vi "DataGenerator.vi"() -> ()   [LabVIEW 2018, in "DataDisplay.lvlib"]
uses:
  DataDisplay.lvlib
  TypeDefine/DD_ChannelInfo.ctl
  <vilib>/measure/NI_MABase.lvlib
panel:
  in  "TrendPlot":bool
  in  "通道信息":T1[](array[typedef])=[{"名称"="位移1", "单位"="mm", "数据类型"=enum."Real", "趋势线"=enum."Y"}, {"名称"="位移2", "单位"="mm", "数据类型"=enum."Real", "趋势线"=enum."Y"}, {"名称"="力1", "单位"="mm", "数据类型"=enum."Real", "趋势线"=enum."N/A"}, {"名称"="力2", "单位"="mm", "数据类型"=enum."Real", "趋势线"=enum."N/A"}, {"名称"="次数1", "单位"="次", "数据类型"=enum."Int", "趋势线"=enum."X"}, {"名称"="次数2", "单位"="次", "数据类型"=enum."Int", "趋势线"=enum."X"}]
  in  "显示采样率":i32=1000
  in  "phase 2":dbl caption="相位" format="%.2p"
  in  "phase":dbl caption="相位" format="%.2p"
  in  "XYPlot":bool
  in  "frequency 2":dbl=10.0 caption="频率" format="%0.2p"
  in  "amplitude 2":dbl=1.0 caption="幅值" format="%0.2p"
  in  "TPlot":bool
  in  "amplitude":dbl=1.0 caption="幅值" format="%0.2p"
  in  "frequency":dbl=10.0 caption="频率" format="%0.2p"
  in  "毫秒倍数":u32=100
  out "Stop":bool
  in  "退出":bool
  in  "数值显示窗":bool
  in  "DD_通道名称列表":string[](array[string])=["位移1", "力1", "次数1", "位移2", "力2", "次数2"]
  in  "原始采样率":i32=10000
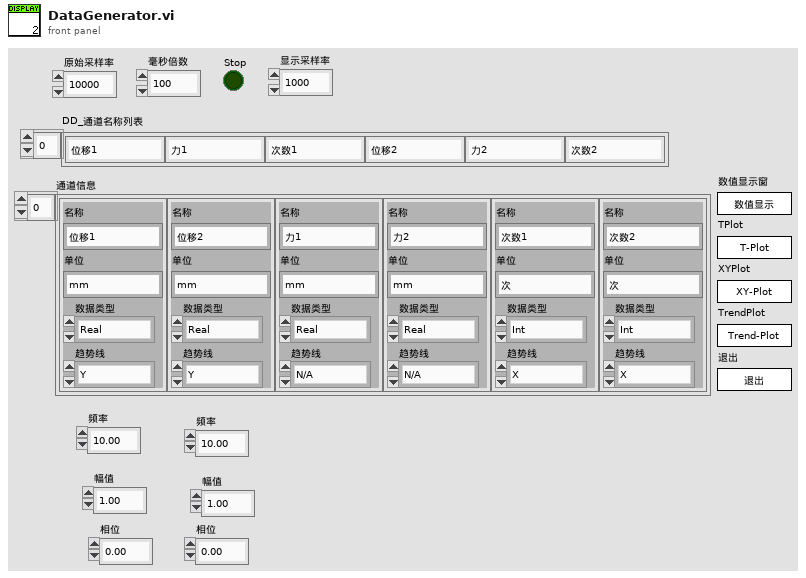
[diagram p1: front panel]
types:
  T1 = typedef "DataDisplay.lvlib/DD_ChannelInfo.ctl" = cluster{"名称":string, "单位":string, "数据类型":enum16{"Real", "Int"}, "趋势线":enum16{"N/A", "X", "Y"}}
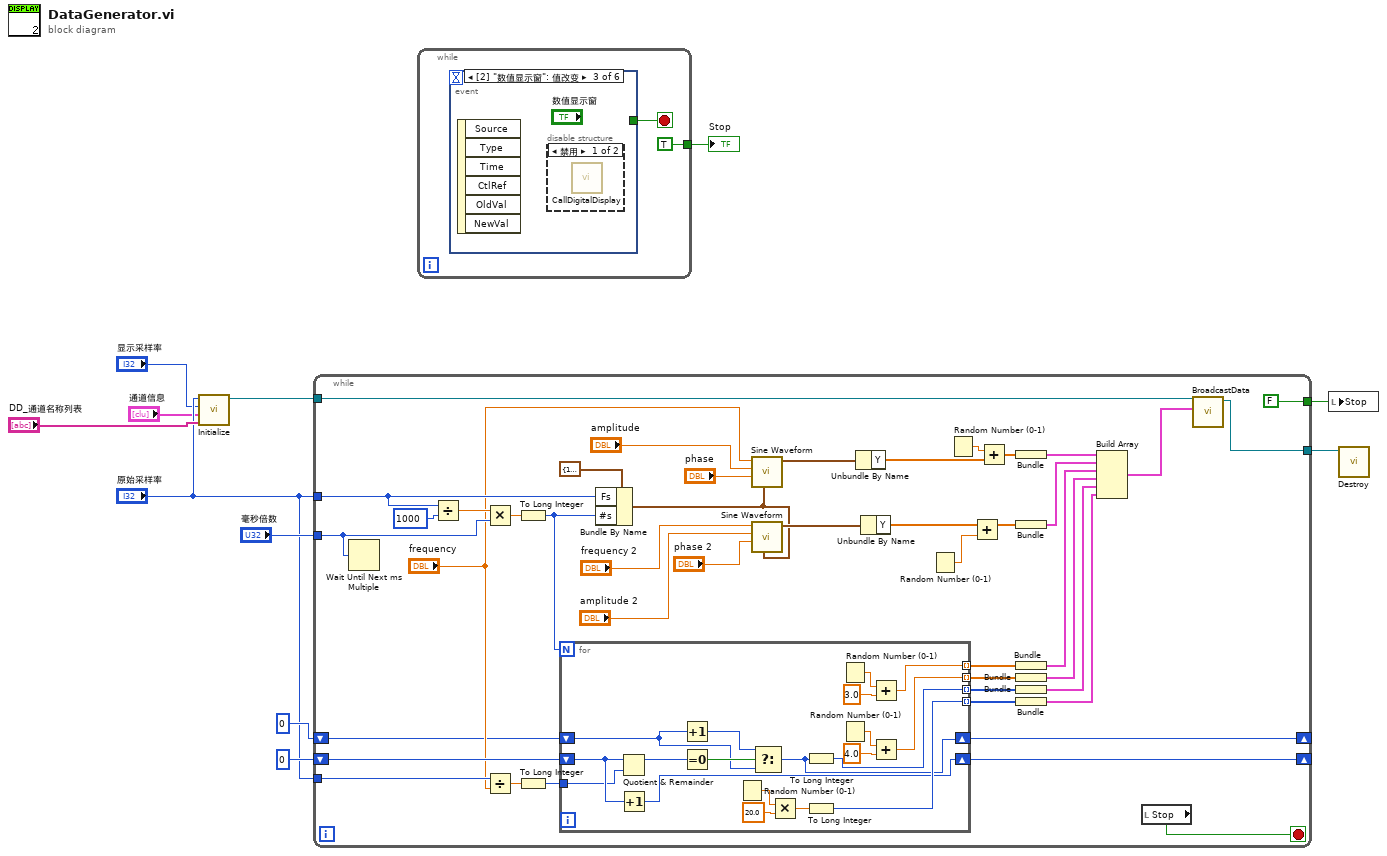
[diagram p0: block diagram]
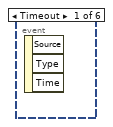
[diagram p2: hidden frame]
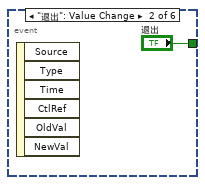
[diagram p3: hidden frame]
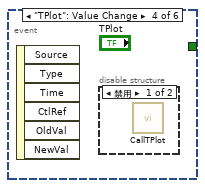
[diagram p5: hidden frame]
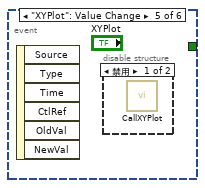
[diagram p7: hidden frame]
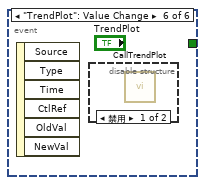
[diagram p9: hidden frame]
diagram:
  n1 = call "Initialize.vi"("DD_通道名称列表"="DD_通道名称列表", "通道信息"="通道信息", "采样率"="显示采样率", "原始采样率"="原始采样率") -> ("通知器输出"=w11:refnum<notifier>)  [unwired: 7 in]
  n2 = while {
    tunnel: w11 -> [w14]
    tunnel: "原始采样率" -> [w38]
    tunnel: [FALSE] -> w9
    tunnel: "毫秒倍数" -> [w40]
    shift-right: [w26] -> _
    shift-left: i64 0 -> [w25]
    tunnel: "原始采样率" -> [w24]
    shift-right: [w19] -> _
    shift-left: 0 -> [w20]
    tunnel: [w12] -> w1
    stop <- w42 stop-if-true
    n3 = Wait Until Next ms Multiple(millisecond multiple=w40) -> ()  [unwired: 1 out]
    n4 = Divide(x=w38, y=1000) -> (x/y=w54:dbl)
    n5 = Multiply(x=w54, y=w40) -> (x*y=w53:dbl)
    n6 = Divide(x=w24, y="frequency") -> (x/y=w22:dbl)
    n7 = To Long Integer(number=w53) -> (32bit integer=w27:i32)
    n8 = To Long Integer(number=w22) -> (32bit integer=w21:i32)
    n9 = for {
      N: w27 -> [_]
      tunnel: [w67] -> w49 mode=indexing
      tunnel: [w66] -> w50 mode=indexing
      tunnel: [w65] -> w51 mode=indexing
      tunnel: [w64] -> w52 mode=indexing
      shift-right: [w63] -> w26
      shift-left: w25 -> [w62]
      tunnel: w21 -> [w61]
      shift-right: [w56] -> w19
      shift-left: w20 -> [w58]
      n10 = Quotient & Remainder(x=w62, y=w61) -> (x-y*floor(x/y)=w60:i64)  [unwired: 1 out]
      n11 = Increment(x=w62) -> (x+1=w63:i64)
      n12 = Increment(x=w58) -> (x+1=w57:i32)
      n13 = Equal To 0?(x=w60) -> (x = 0?=w59:bool)
      n14 = Random Number (0-1)() -> (number: 0 to 1=w70:dbl)
      n15 = Select(t=w57, s=w59, f=w58) -> (s? t:f=w56:i32)
      n16 = Multiply(x=w70, y=20.0) -> (x*y=w68:dbl)
      n17 = To Long Integer(number=w56) -> (32bit integer=w65:i32)
      n18 = To Long Integer(number=w68) -> (32bit integer=w64:i32)
      n19 = Random Number (0-1)() -> (number: 0 to 1=w74:dbl)
      n20 = Random Number (0-1)() -> (number: 0 to 1=w73:dbl)
      n21 = Add(x=w74, y=3.0) -> (x+y=w67:dbl)
      n22 = Add(x=w73, y=4.0) -> (x+y=w66:dbl)
    }
    n23 = Bundle By Name(cluster=cluster{"Fs":dbl, "#s":dbl} {"Fs"=1000.0, "#s"=1000.0} ("sampling info"), "Fs"=w38, "#s"=w27) -> (w31:cluster{"Fs":dbl, "#s":dbl})
    n24 = call <vilib>:"Sine Waveform.vi"("sampling info"=w31, "phase"="phase", "amplitude"="amplitude", "frequency"="frequency") -> ("signal out"=w37:waveform(dbl))  [unwired: 6 in, 1 out]
    n25 = call <vilib>:"Sine Waveform.vi"("sampling info"=w31, "phase"="phase 2", "amplitude"="amplitude 2", "frequency"="frequency 2") -> ("signal out"=w32:waveform(dbl))  [unwired: 6 in, 1 out]
    n26 = Unbundle By Name(w37) -> ("Y"=w36:dbl[])
    n27 = Unbundle By Name(w32) -> ("Y"=w30:dbl[])
    n28 = Random Number (0-1)() -> (number: 0 to 1=w15:dbl)
    n29 = Random Number (0-1)() -> (number: 0 to 1=w17:dbl)
    n30 = Add(x=w30, y=w15) -> (x+y=w16:dbl[])
    n31 = Add(x=w17, y=w36) -> (x+y=w18:dbl[])
    n32 = Bundle(w18) -> (w48:cluster{dbl[]})  [unwired: 1 in]
    n33 = Bundle(w16) -> (w47:cluster{dbl[]})  [unwired: 1 in]
    n34 = Bundle(w49) -> (w46:cluster{dbl[]})  [unwired: 1 in]
    n35 = Bundle(w50) -> (w45:cluster{dbl[]})  [unwired: 1 in]
    n36 = Bundle(w51) -> (w44:cluster{i32[]})  [unwired: 1 in]
    n37 = Bundle(w52) -> (w43:cluster{i32[]})  [unwired: 1 in]
    n38 = Build Array(w48, w47, w46, w45, w44, w43) -> (w13:cluster{dbl[]}[])
    n39 = local read "Stop"() -> (w42:bool)
    n40 = call "BroadcastData.vi"("Data"=w13, "通知器输入"=w14) -> ("通知器输出"=w12:refnum<notifier>)  [unwired: 9 in]
  }
  n41 = while {
    tunnel: [TRUE] -> w10
    stop <- w76 stop-if-true
    n42 = event shown="[2] \"数值显示窗\": 值改变" {
      selector: _ -> [_ _ _ _ _ _]
      dyn-events: _ -> [_ _ _ _ _ _]
      timeout: _ -> [_ _ _ _ _ _]
      tunnel: [_ "退出" _ _ _ _] -> w76
      event Timeout {
        n43 = event-data() -> ()  [unwired: 1 in, 3 out]
      }
      event "退出": Value Change {
        n44 = event-data() -> ()  [unwired: 1 in, 6 out]
      }
      event "数值显示窗": Value Change {
        n45 = event-data() -> ()  [unwired: 1 in, 6 out]
        n46 = disable-structure shown="禁用" {
          frame Disabled {
            n47 = call "CallDigitalDisplay.vi"() -> ()  [unwired: 11 in, 1 out]
          }
          frame Enabled {
          }
        }
      }
      event "TPlot": Value Change {
        n48 = event-data() -> ()  [unwired: 1 in, 6 out]
        n49 = disable-structure shown="禁用" {
          frame Disabled {
            n50 = call "CallTPlot.vi"() -> ()  [unwired: 10 in, 2 out]
          }
          frame Enabled {
          }
        }
      }
      event "XYPlot": Value Change {
        n51 = event-data() -> ()  [unwired: 1 in, 6 out]
        n52 = disable-structure shown="禁用" {
          frame Disabled {
            n53 = call "CallXYPlot.vi"() -> ()  [unwired: 10 in, 2 out]
          }
          frame Enabled {
          }
        }
      }
      event "TrendPlot": Value Change {
        n54 = event-data() -> ()  [unwired: 1 in, 6 out]
        n55 = disable-structure shown="禁用" {
          frame Disabled {
            n56 = call "CallTrendPlot.vi"() -> ()  [unwired: 10 in, 2 out]
          }
          frame Enabled {
          }
        }
      }
    }
  }
  "Stop" <- w10
  n57 = local write "Stop"(w9) -> ()
  n58 = call "Destroy.vi"("通知器输入"=w1) -> ()  [unwired: 10 in, 1 out]
